vi "Administration.vi"() -> ()   [LabVIEW 2017]
uses:
  admin_settings.vi
  <vilib>/Utility/config.llb/Write Key (Double).vi
  <vilib>/Utility/config.llb/Write Key (Boolean).vi
  <vilib>/Utility/config.llb/Write Key (String).vi
  <vilib>/Utility/config.llb/NI_LVConfig.lvlib
panel:
  out "password":string
  out "user":string
  in  "Login data":cluster{"user":string, "password":string}
  out "NI 2":i64 format="%x"
  out "NI 1":i64 format="%x"
  in  "Apply":bool
  out "String":string
  in  "Testing Mode":bool
  in  "NI Devices Serial Number":cluster{"NI 1":i64, "NI 2":i64}={"NI 1"=30585608, "NI 2"=30585101}
  in  "close":bool
  # "Administration Panel"
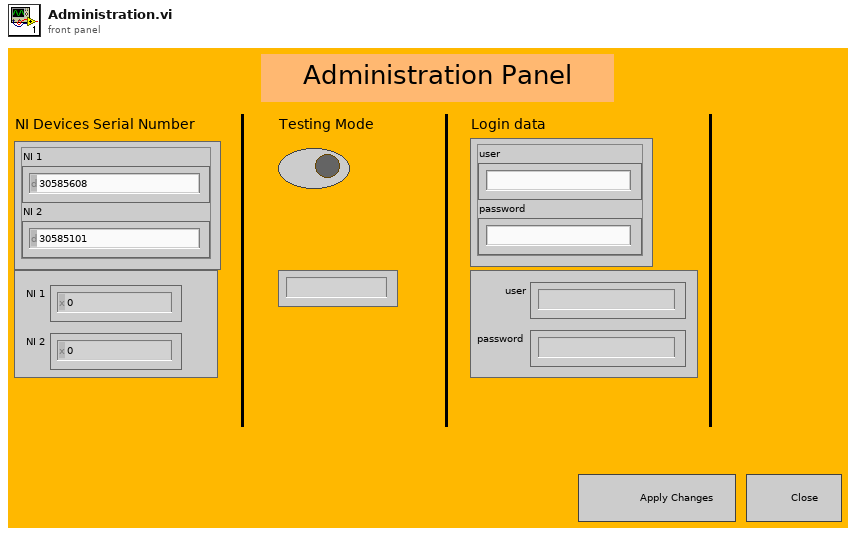
[diagram p1: front panel]
types:
  T1 = typedef "NI_LVConfig.lvlib/Config Data RefNum.ctl" = refnum<k1>
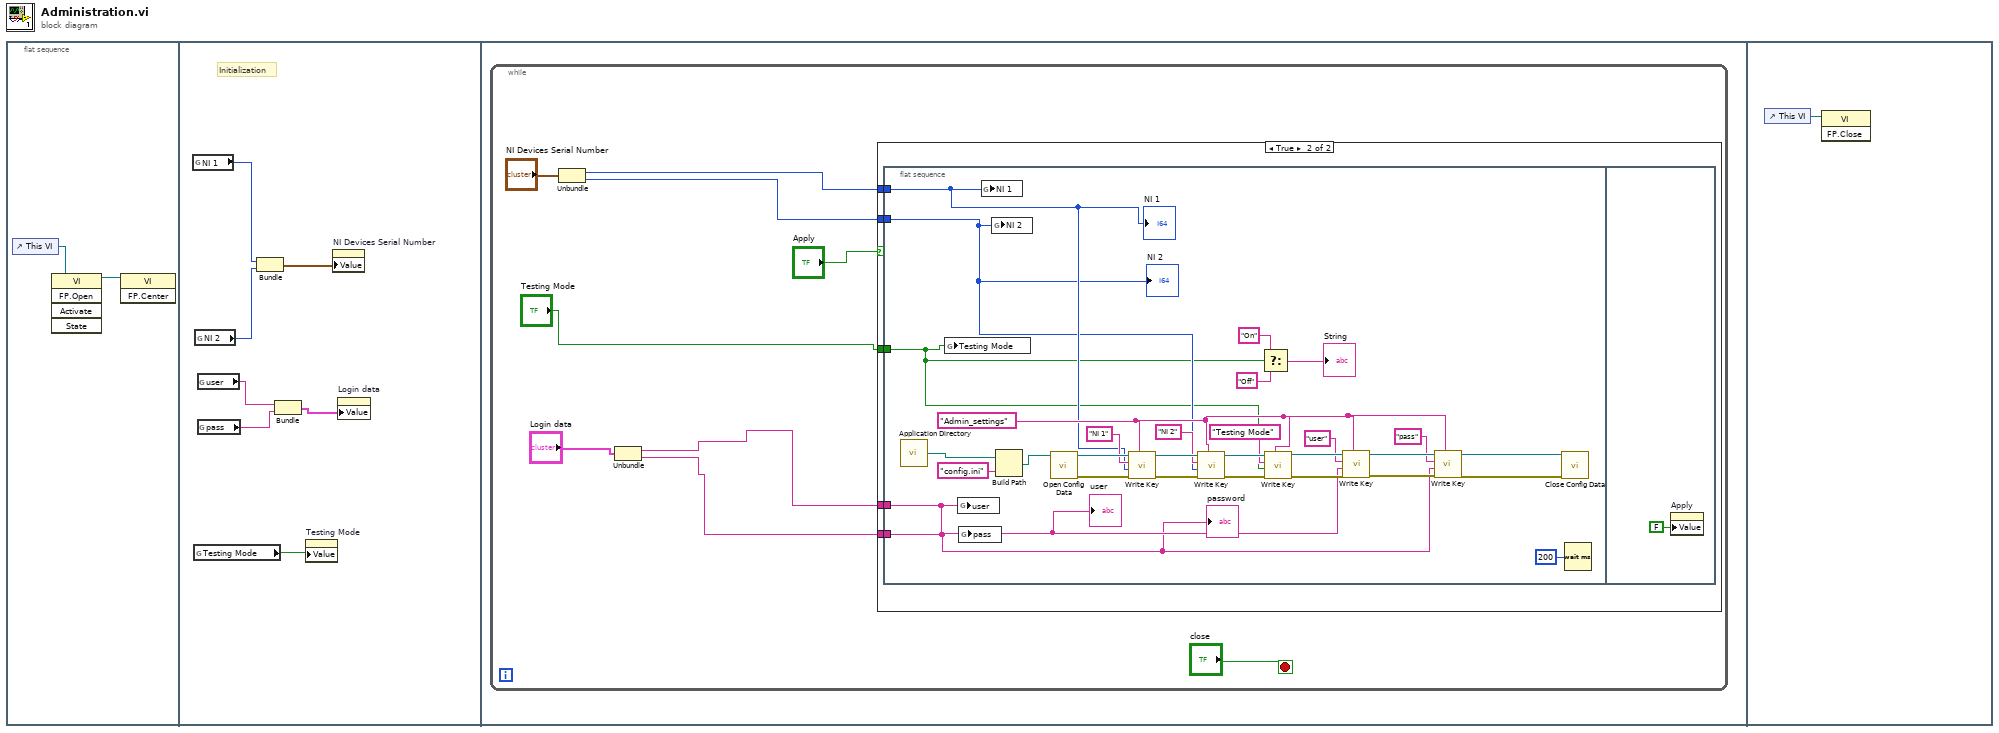
[diagram p0: block diagram]
diagram:
  n1 = flat-sequence {
    frame #0 {
      n2 = control-ref of="This VI"() -> (w2:refnum<vi>)
      n3 = invoke class="VI" method="FP.Open"(reference=w2) -> (reference out=w1:refnum<vi>)  [unwired: 4 in, 4 out]
      n4 = invoke class="VI" method="FP.Center"(reference=w1) -> ()  [unwired: 2 in, 3 out]
    }
    frame #1 {
      # "Initialization"
      n5 = global read "admin_settings.vi" "NI 1"() -> (w9:i64)
      n6 = global read "admin_settings.vi" "Testing Mode"() -> (w6:bool)
      n7 = global read "admin_settings.vi" "NI 2"() -> (w8:i64)
      n8 = global read "admin_settings.vi" "user"() -> (w5:string)
      n9 = global read "admin_settings.vi" "pass"() -> (w4:string)
      n10 = Bundle("NI 1"=w9, "NI 2"=w8) -> (w7:cluster{"NI 1":i64, "NI 2":i64})  [unwired: 1 in]
      n11 = Bundle("user"=w5, "pass"=w4) -> (w3:cluster{"user":string, "pass":string})  [unwired: 1 in]
      n12 = property on="Testing Mode" class="Bool (strict)"("Value"=w6) -> ()  [unwired: 2 in, 2 out]
      n13 = property on="NI Devices Serial Number" class="Clust (strict)"("Value"=w7) -> ()  [unwired: 2 in, 2 out]
      n14 = property on="Login data" class="Clust (strict)"("Value"=w3) -> ()  [unwired: 2 in, 2 out]
    }
    frame #2 {
      n15 = while {
        stop <- "close" stop-if-true
        n16 = Unbundle("NI Devices Serial Number") -> ("NI 1"=w15:i64, "NI 2"=w14:i64)
        n17 = Unbundle("Login data") -> ("user"=w12:string, "password"=w11:string)
        n18 = case shown="True" "Apply" {
          tunnel: w15 -> [_ w23]
          tunnel: w14 -> [_ w22]
          tunnel: "Testing Mode" -> [_ w21]
          tunnel: w12 -> [_ w20]
          tunnel: w11 -> [_ w19]
          frame False {
          }
          frame True {
            n19 = flat-sequence {
              tunnel: w23 -> [w31]
              tunnel: w22 -> [w30]
              tunnel: w21 -> [w26]
              tunnel: w20 -> [w25]
              tunnel: w19 -> [w24]
              frame #0 {
                w34 = "Admin_settings" ("section")
                n20 = call <vilib>:"Application Directory.vi"() -> ("Application Directory"=w52:path)
                n21 = global write "admin_settings.vi" "Testing Mode"(w26) -> ()
                n22 = global write "admin_settings.vi" "user"(w25) -> ()
                n23 = global write "admin_settings.vi" "pass"(w24) -> ()
                n24 = global write "admin_settings.vi" "NI 1"(w31) -> ()
                n25 = global write "admin_settings.vi" "NI 2"(w30) -> ()
                n26 = Build Path(base path=w52, name or relative path="config.ini") -> (appended path=w51:path)
                n27 = call <vilib>:"Open Config Data.vi"("configuration file path"=w51) -> ("error out"=w47:errorcluster, "refnum"=w50:T1)  [unwired: 8 in, 1 out]
                n28 = call-poly <vilib>:"Write Key.vi"("section"=w34, "error in (no error)"=w47, "value"=w31, "key"="NI 1", "refnum"=w50) -> ("error out"=w46:errorcluster, "refnum out"=w49:T1)  [unwired: 4 in, 1 out]
                n29 = call-poly <vilib>:"Write Key.vi"("section"=w34, "error in (no error)"=w46, "value"=w30, "key"="NI 2", "refnum"=w49) -> ("error out"=w45:errorcluster, "refnum out"=w48:T1)  [unwired: 4 in, 1 out]
                n30 = Select(t="On", s=w26, f="Off") -> (s? t:f=→"String":string)
                n31 = call-poly <vilib>:"Write Key.vi"("section"=w34, "error in (no error)"=w45, "value"=w26, "key"="Testing Mode", "refnum"=w48) -> ("error out"=w36:errorcluster, "refnum out"=w37:T1)  [unwired: 4 in, 1 out]
                n32 = call-poly <vilib>:"Write Key.vi"("section"=w34, "error in (no error)"=w36, "value"=w25, "key"="user", "refnum"=w37) -> ("error out"=w35:errorcluster, "refnum out"=w38:T1)  [unwired: 4 in, 1 out]
                n33 = call-poly <vilib>:"Write Key.vi"("section"=w34, "error in (no error)"=w35, "value"=w24, "key"="pass", "refnum"=w38) -> ("error out"=w39:errorcluster, "refnum out"=w40:T1)  [unwired: 4 in, 1 out]
                n34 = call <vilib>:"Close Config Data.vi"("error in (no error)"=w39, "refnum"=w40) -> ()  [unwired: 8 in, 2 out]
                n35 = Wait (ms)(milliseconds to wait=u32 200) -> ()  [unwired: 1 out]
                "NI 1" <- w31
                "NI 2" <- w30
                "user" <- w25
                "password" <- w24
              }
              frame #1 {
                n36 = property on="Apply" class="Bool (strict)"("Value"=FALSE ("Apply")) -> ()  [unwired: 2 in, 2 out]
              }
            }
          }
        }
      }
    }
    frame #3 {
      n37 = control-ref of="This VI"() -> (w55:refnum<vi>)
      n38 = invoke class="VI" method="FP.Close"(reference=w55) -> ()  [unwired: 2 in, 3 out]
    }
  }
